vi "compare_file2MK.vi"(8 "Fehler (Eingang, kein Fehler)":errorcluster, 10 "ModuleKindIndex":i32, 11 "Pfad":path) -> (0 "error out":errorcluster, 3 "file=module":bool)   [LabVIEW 2016]
uses:
  <vilib>/Utility/config.llb/Read Key (I32).vi
  <vilib>/Utility/config.llb/NI_LVConfig.lvlib
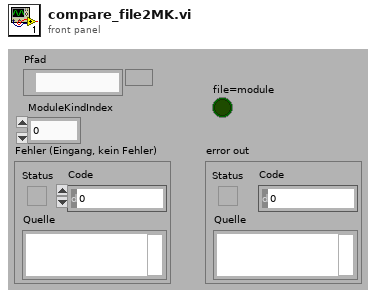
[diagram p1: front panel]
types:
  T1 = typedef "NI_LVConfig.lvlib/Config Data RefNum.ctl" = refnum<k1>
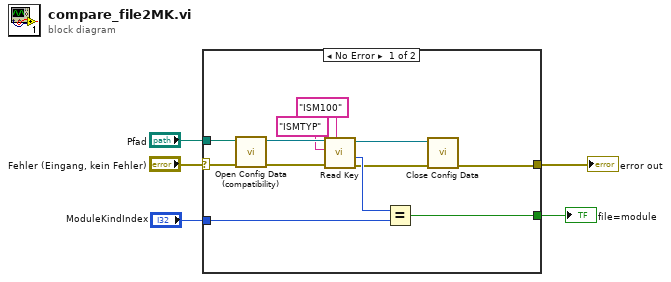
[diagram p0: block diagram]
diagram:
  n1 = case shown="No Error" "Fehler (Eingang, kein Fehler)" {
    selector: "Fehler (Eingang, kein Fehler)" -> [w17 w18]
    tunnel: [w6 w18] -> w4
    tunnel: "Pfad" -> [w16 _]
    tunnel: "ModuleKindIndex" -> [w10 _]
    tunnel: [w7 _] -> w1
    frame No Error {
      n2 = call <vilib>:"Open Config Data (compatibility).vi"("error in (no error)"=w17, "configuration file path"=w16) -> ("error out"=w12:errorcluster, "refnum"=w15:T1)  [unwired: 7 in, 1 out]
      n3 = call-poly <vilib>:"Read Key.vi"("section"="ISM100", "error in (no error)"=w12, "key"="ISMTYP", "refnum"=w15) -> ("error out"=w8:errorcluster, "value"=w11:i32, "refnum out"=w9:T1)  [unwired: 4 in, 1 out]
      n4 = Equal?(x=w11, y=w10) -> (x = y?=w7:bool)
      n5 = call <vilib>:"Close Config Data.vi"("error in (no error)"=w8, "refnum"=w9) -> ("error out"=w6:errorcluster)  [unwired: 1 in, 8 out]
    }
    frame Error {
    }
  }
  "error out" <- w4
  "file=module" <- w1
